vi "SR1.destructor.vi"(0 "i ref in":refnum<vi>, 5 "error in (no error)":errorcluster) -> (19 "error out":errorcluster)   [LabVIEW 2014, in "SR1.lvlib"]
doc: "This is the destructor of a class.\n\nLicense Agreement for this software:\n\nCopyright (C)\nGesellschaft für Schwerionenforschung, GSI\nPlanckstr. 1\n64291 Darmstadt\nGermany\n\nContact: D.Beck@gsi.de \n\nThis program is free software; you can redistribute it and/or modify it under the terms of the \nGNU General Public License as published by the Free Software Foundation; either version 2 of \nthe license, or (at your option) any later version.\n\nThis program is distributed in the hope that it will be useful, but WITHOUT ANY WARRANTY; \nwithout even the implied warranty of MERCHANTABILITY or FITNESS FOR A PARTICULAR PURPOSE. See the GNU General License for more details (http://www.gnu.org).\n\nGesellschaft für Schwerionenforschung, GSI\nPlanckstr. 1, 64291 Darmstadt, Germany\nFor all questions and ideas contact: M.Richter@gsi.de, H.Brand@gsi.de or D.Beck@gsi.de.\nLast update: 16-JUN-2004"
uses:
  SR1.lvlib
  CS_Core/CSApplicationBaseClasses/MCSBase/MCSBase.lvlib
  CS_Core/CSApplicationBaseClasses/NABase/NABase.lvlib
  instr.lib/Stanford Research SR1/Stanford Research SR1.lvlib
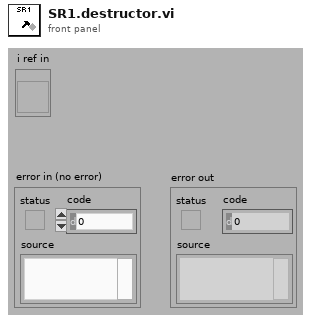
[diagram p1: front panel]
types:
  T1 = enum16{"SetAttribute", "GetAttribute", "CreateAttribute", "DestroyAttribute", "DestroyAllAtributes"}
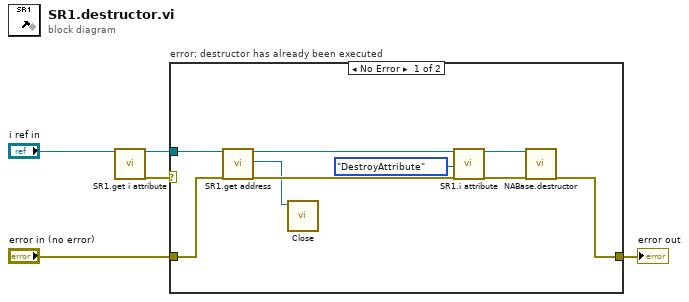
[diagram p0: block diagram]
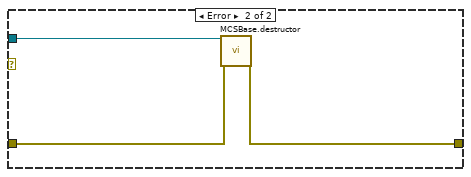
[diagram p2: hidden frame]
diagram:
  n1 = call "SR1.get i attribute.vi"("i ref in"="i ref in") -> ("i ref out"=w1:refnum<vi>, "error out"=w2:errorcluster)  [unwired: 16 in, 1 out]
  n2 = case "error: destructor has already been executed" shown="No Error" w2 {
    tunnel: [w11 w15] -> w5
    tunnel: "error in (no error)" -> [w9 w16]
    tunnel: w1 -> [w10 w17]
    frame No Error {
      n3 = call "SR1.get address.vi"("i ref in"=w10, "error in (no error)"=w9) -> ("i ref out"=w7:refnum<vi>, "VISA resource name"=w6:refnum<visa-resource-name>, "error out"=w8:errorcluster)  [unwired: 15 in]
      n4 = call "Close.vi"("VISA resource name"=w6) -> ()  [unwired: 10 in, 1 out]
      n5 = call "SR1.i attribute.vi"("VI Refnum"=w7, "Action"=T1."DestroyAttribute", "error in (no error)"=w8) -> ("VI Refnum out"=w13:refnum<vi>, "error out"=w12:errorcluster)  [unwired: 14 in, 1 out]
      n6 = call "NABase.destructor.vi"("i ref in"=w13, "error in (no error)"=w12) -> ("error out"=w11:errorcluster)  [unwired: 17 in]
    }
    frame Error {
      n7 = call "MCSBase.destructor.vi"("i ref in"=w17, "error in (no error)"=w16) -> ("error out"=w15:errorcluster)  [unwired: 17 in]
    }
  }
  "error out" <- w5
